vi "LockinVsgGraphs.vi"(7 "reset?":bool, 10 "paramter in":dbl, 11 "Y array in":dbl[](array[numeric])) -> (2 "Y vs X":cluster{"Y":dbl[], "Y":dbl[]}[](array[cluster]), 3 "Array out":cluster{"Y":dbl[], "Y":dbl[]}[](array[cluster]))   [LabVIEW 2016, in "Transport.lvclass"]
uses:
  Transport.lvclass
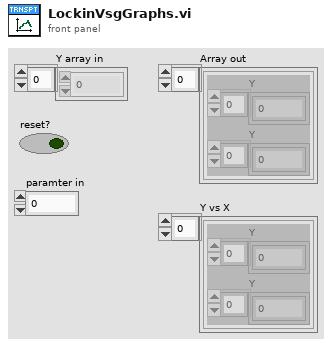
[diagram p1: front panel]
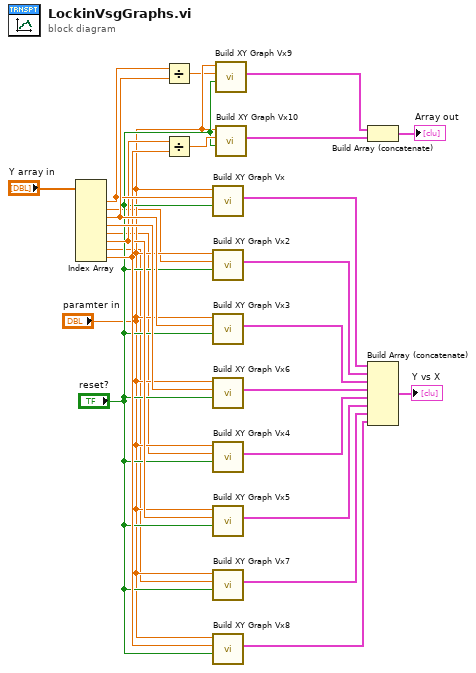
[diagram p0: block diagram]
diagram:
  n1 = Index Array(array="Y array in") -> (element #1=w19:dbl, element #2=w3:dbl, element #3=w21:dbl, element #4=w20:dbl, element #5=w4:dbl, element #6=w13:dbl, element #7=w8:dbl, element #8=w14:dbl)  [unwired: 8 in]
  n2 = Divide(x=w19, y=w21) -> (x/y=w10:dbl)
  n3 = Divide(x=w13, y=w14) -> (x/y=w15:dbl)
  n4 = call "Build XY Graph Vx"("Reset"="reset?", "Y Input"=w19, "X Input"="paramter in") -> ("XY Graph"=w1:cluster{"Y":dbl[], "Y":dbl[]}[])  [unwired: 2 in, 6 out]
  n5 = call "Build XY Graph Vx2"("Reset"="reset?", "Y Input"=w3, "X Input"="paramter in") -> ("XY Graph"=w2:cluster{"Y":dbl[], "Y":dbl[]}[])  [unwired: 2 in, 6 out]
  n6 = call "Build XY Graph Vx3"("Reset"="reset?", "Y Input"=w21, "X Input"="paramter in") -> ("XY Graph"=w24:cluster{"Y":dbl[], "Y":dbl[]}[])  [unwired: 2 in, 6 out]
  n7 = call "Build XY Graph Vx6"("Reset"="reset?", "Y Input"=w20, "X Input"="paramter in") -> ("XY Graph"=w23:cluster{"Y":dbl[], "Y":dbl[]}[])  [unwired: 2 in, 6 out]
  n8 = call "Build XY Graph Vx4"("Reset"="reset?", "Y Input"=w4, "X Input"="paramter in") -> ("XY Graph"=w25:cluster{"Y":dbl[], "Y":dbl[]}[])  [unwired: 2 in, 6 out]
  n9 = call "Build XY Graph Vx5"("Reset"="reset?", "Y Input"=w13, "X Input"="paramter in") -> ("XY Graph"=w5:cluster{"Y":dbl[], "Y":dbl[]}[])  [unwired: 2 in, 6 out]
  n10 = call "Build XY Graph Vx7"("Reset"="reset?", "Y Input"=w8, "X Input"="paramter in") -> ("XY Graph"=w6:cluster{"Y":dbl[], "Y":dbl[]}[])  [unwired: 2 in, 6 out]
  n11 = call "Build XY Graph Vx8"("Reset"="reset?", "Y Input"=w14, "X Input"="paramter in") -> ("XY Graph"=w7:cluster{"Y":dbl[], "Y":dbl[]}[])  [unwired: 2 in, 6 out]
  n12 = call "Build XY Graph Vx9"("Reset"="reset?", "Y Input"=w10, "X Input"="paramter in") -> ("XY Graph"=w16:cluster{"Y":dbl[], "Y":dbl[]}[])  [unwired: 2 in, 6 out]
  n13 = call "Build XY Graph Vx10"("Reset"="reset?", "Y Input"=w15, "X Input"="paramter in") -> ("XY Graph"=w17:cluster{"Y":dbl[], "Y":dbl[]}[])  [unwired: 2 in, 6 out]
  n14 = Build Array (concatenate)(w16, w17) -> (→"Array out":cluster{"Y":dbl[], "Y":dbl[]}[])
  n15 = Build Array (concatenate)(w1, w2, w24, w23, w25, w5, w6, w7) -> (→"Y vs X":cluster{"Y":dbl[], "Y":dbl[]}[])
